vi "Read Value.vi"(11 "TestManagerMsg.Measurement in":refnum<class "TestManagerMsg.Measurement.lvclass">) -> (2 "Value":variant, 3 "TestManagerMsg.Measurement out":refnum<class "TestManagerMsg.Measurement.lvclass">)   [LabVIEW 2020, in "Caraya.lvlib" / "TestManagerMsg.Measurement.lvclass"]
uses:
  TestManagerMsg.Measurement.lvclass
  TestManagerMsg.Measurement.lvclass/TestManagerMsg.Measurement.ctl
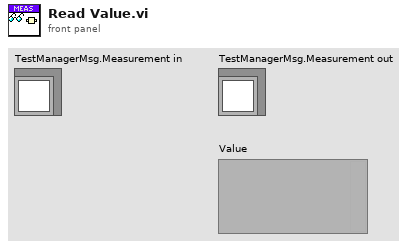
[diagram p1: front panel]
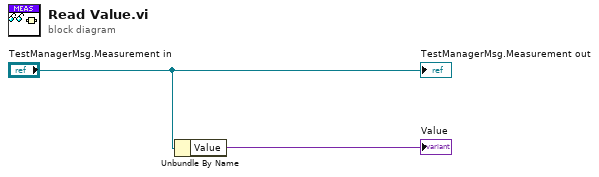
[diagram p0: block diagram]
diagram:
  n1 = Unbundle By Name("TestManagerMsg.Measurement in") -> ("Value"=→"Value":variant)
  "TestManagerMsg.Measurement out" <- "TestManagerMsg.Measurement in"
